vi "Path 2.vi"() -> (3 "appended path":path)   [LabVIEW 2014]
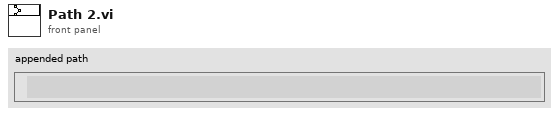
[diagram p1: front panel]
types:
  T1 = enum32{"invalid app kind", "Development System", "Run Time System", "Student Edition", "Embedded LabVIEW", "Evaluation", "Custom"}
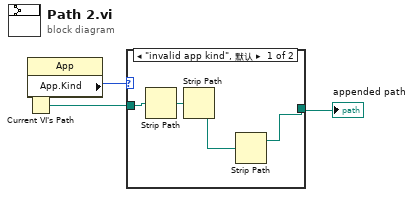
[diagram p0: block diagram]
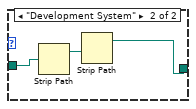
[diagram p2: hidden frame]
diagram:
  n1 = Current VI's Path() -> (path=w2:path)
  n2 = property class="App"() -> ("App.Kind"=w1:T1)  [unwired: 2 in, 2 out]
  n3 = case shown="\"invalid app kind\", 默认" w1 {
    tunnel: w2 -> [w7 w10]
    tunnel: [w4 w8] -> w3
    frame "invalid app kind", Default {
      n4 = Strip Path(path=w7) -> (stripped path=w6:path)  [unwired: 1 out]
      n5 = Strip Path(path=w6) -> (stripped path=w5:path)  [unwired: 1 out]
      n6 = Strip Path(path=w5) -> (stripped path=w4:path)  [unwired: 1 out]
    }
    frame "Development System" {
      n7 = Strip Path(path=w10) -> (stripped path=w9:path)  [unwired: 1 out]
      n8 = Strip Path(path=w9) -> (stripped path=w8:path)  [unwired: 1 out]
    }
  }
  "appended path" <- w3
